vi "AutoConfigPlots.vi"(8 "LineWidth":u8, 9 "Y标尺总数":i32, 10 "已选信号数组":refnum<vi>, 11 "XYGraph输入":refnum<vi>) -> ()   [LabVIEW 2015]
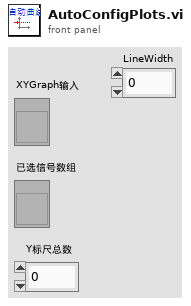
[diagram p1: front panel]
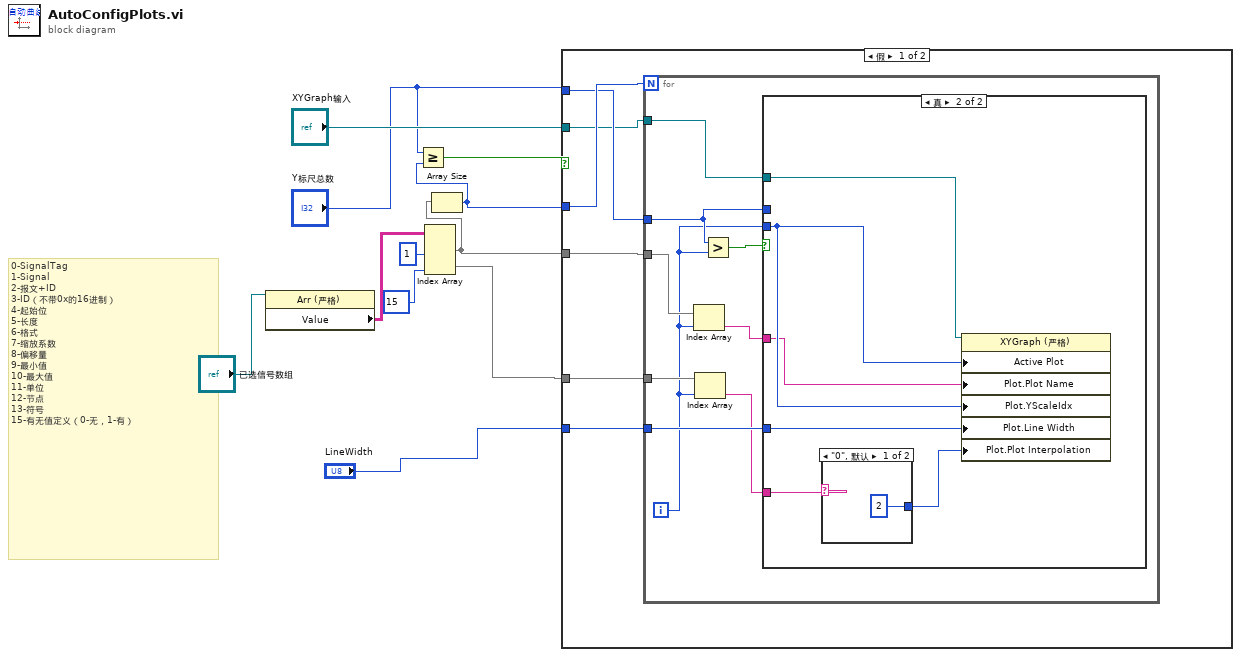
[diagram p0: block diagram]
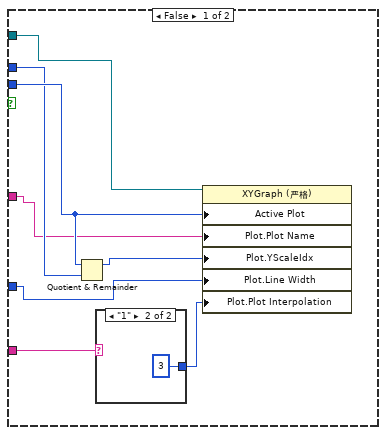
[diagram p2: hidden frame]
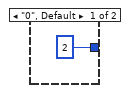
[diagram p3: hidden frame]
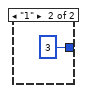
[diagram p4: hidden frame]
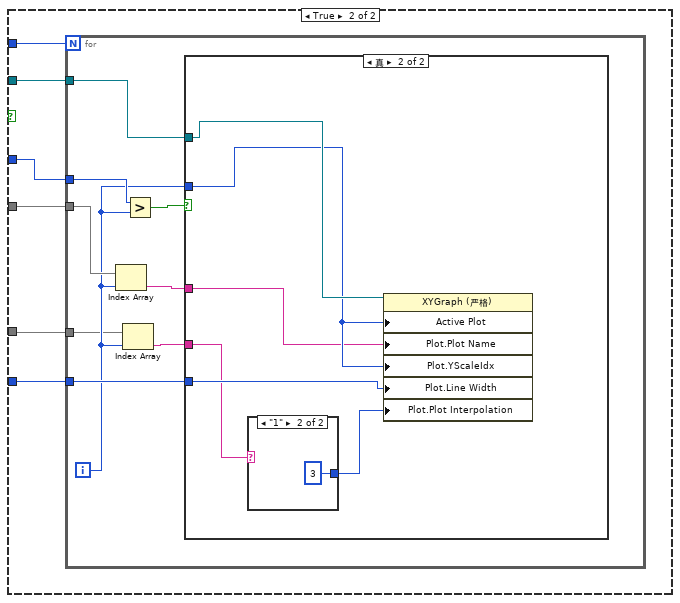
[diagram p5: hidden frame]
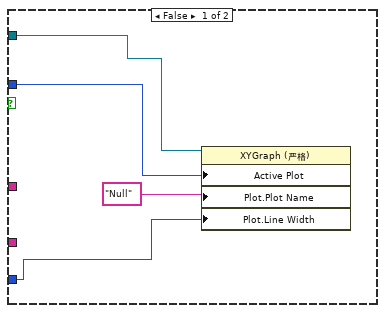
[diagram p6: hidden frame]
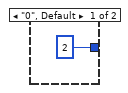
[diagram p7: hidden frame]
diagram:
  # "0-SignalTag\n1-Signal\n2-报文+ID\n3-ID（不带0x的16进制）\n4-起始位\n5-长度\n6-格式\n7-缩放系数\n8-偏移量\n9-最小值\n10-最大值\n11-单位\n12-节点\n13-符号\n15-有无值定义（0-无，1-有）"
  n1 = property class="Arr (严格)"(reference="已选信号数组") -> ("Value"=w5:string[][])  [unwired: 1 in, 2 out]
  n2 = Index Array(array=w5, index (col) #1=1 ("禁用的索引 (列)"), index (col) #2=15 ("索引 (列)")) -> (element #1=w9:string[], element #2=w1:string[])  [unwired: 2 in]
  n3 = Array Size(array=w9) -> (size(s)=w10:i32)
  n4 = Greater Or Equal?(x="Y标尺总数", y=w10) -> (x >= y?=w7:bool)
  n5 = case shown="假" w7 {
    tunnel: "Y标尺总数" -> [w15 w50]
    tunnel: w9 -> [w17 w49]
    tunnel: w10 -> [w16 w48]
    tunnel: "XYGraph输入" -> [w14 w47]
    tunnel: "LineWidth" -> [w13 w46]
    tunnel: w1 -> [w12 w45]
    frame False {
      n6 = for {
        N: w16 -> [_]
        tunnel: w17 -> [w24]
        tunnel: w15 -> [w22]
        tunnel: w14 -> [w23]
        tunnel: w13 -> [w21]
        tunnel: w12 -> [w20]
        i -> [w19]
        n7 = Index Array(array=w24, index=w19) -> (element=w25:string)
        n8 = Index Array(array=w20, index=w19) -> (element=w18:string)
        n9 = Greater?(x=w22, y=w19) -> (0:w26:bool)
        n10 = case shown="真" w26 {
          tunnel: w23 -> [w34 w42]
          tunnel: w19 -> [w33 w41]
          tunnel: w25 -> [w31 w40]
          tunnel: w22 -> [w32 _]
          tunnel: w21 -> [w29 w39]
          tunnel: w18 -> [w28 w38]
          frame False {
            n11 = Quotient & Remainder(x=w33, y=w32) -> (x-y*floor(x/y)=w30:i32)  [unwired: 1 out]
            n12 = case shown="\"1\"" w28 {
              tunnel: [u8 2 ("曲线.曲线插值") u8 3 ("曲线.曲线插值")] -> w27
              frame "0", Default {
              }
              frame "1" {
              }
            }
            n13 = property class="XYGraph (严格)"(reference=w34, "Active Plot"=w33, "Plot.Plot Name"=w31, "Plot.YScaleIdx"=w30, "Plot.Line Width"=w29, "Plot.Plot Interpolation"=w27) -> ()  [unwired: 1 in, 2 out]
          }
          frame True {
            n14 = case shown="\"0\", 默认" w38 {
              tunnel: [u8 2 ("曲线.曲线插值") u8 3 ("曲线.曲线插值")] -> w37
              frame "0", Default {
              }
              frame "1" {
              }
            }
            n15 = property class="XYGraph (严格)"(reference=w42, "Active Plot"=w41, "Plot.Plot Name"=w40, "Plot.YScaleIdx"=w41, "Plot.Line Width"=w39, "Plot.Plot Interpolation"=w37) -> ()  [unwired: 1 in, 2 out]
          }
        }
      }
    }
    frame True {
      n16 = for {
        N: w50 -> [_]
        tunnel: w49 -> [w57]
        tunnel: w48 -> [w56]
        tunnel: w47 -> [w55]
        tunnel: w46 -> [w54]
        tunnel: w45 -> [w52]
        i -> [w53]
        n17 = Index Array(array=w57, index=w53) -> (element=w58:string)
        n18 = Index Array(array=w52, index=w53) -> (element=w51:string)
        n19 = Greater?(x=w56, y=w53) -> (0:w59:bool)
        n20 = case shown="真" w59 {
          tunnel: w55 -> [w63 w69]
          tunnel: w53 -> [w61 w68]
          tunnel: w58 -> [_ w67]
          tunnel: w54 -> [w60 w66]
          tunnel: w51 -> [_ w65]
          frame False {
            n21 = property class="XYGraph (严格)"(reference=w63, "Active Plot"=w61, "Plot.Plot Name"="Null" ("曲线.曲线名"), "Plot.Line Width"=w60) -> ()  [unwired: 1 in, 2 out]
          }
          frame True {
            n22 = case shown="\"1\"" w65 {
              tunnel: [u8 2 ("曲线.曲线插值") u8 3 ("曲线.曲线插值")] -> w64
              frame "0", Default {
              }
              frame "1" {
              }
            }
            n23 = property class="XYGraph (严格)"(reference=w69, "Active Plot"=w68, "Plot.Plot Name"=w67, "Plot.YScaleIdx"=w68, "Plot.Line Width"=w66, "Plot.Plot Interpolation"=w64) -> ()  [unwired: 1 in, 2 out]
          }
        }
      }
    }
  }
